vi "Acq 3.5 RT.vi"() -> ()   [LabVIEW 2021]
uses:
  <vilib>/FPGAPlugInAG/myRIO-1900/niLvFpga_Open_myRIO-1900.vi
  <vilib>/rvi/interface/common/dynamic/niFpgaDynamicAddResources.vi
  <vilib>/rvi/interface/common/niFpgaWaitOnOcc.vi
  <vilib>/Utility/error.llb/Error Cluster From Error Code.vi
  <vilib>/rvi/errors/niLvFpgaAdjustHostInterfaceError.vi
  <vilib>/FPGAPlugInAG/Dynamic/niLvFpga_Close_Dynamic.vi
  <vilib>/rvi/interface/nirviOpenFPGA/nirviOpenFPGA.xnode
  FPGA Bitfiles/acquisition3.5co_FPGATarget_Acq3.5FPGA_iMy6CG-4QfE.lvbitx
  <vilib>/rvi/interface/nirviMethod/nirviMethod.xnode
  <vilib>/rvi/interface/nirviReadWriteControl/nirviReadWriteControl.xnode
  <vilib>/rvi/interface/nirviCloseFPGA/nirviCloseFPGA.xnode
  <vilib>/rvi/errors/niLvFpgaMergeErrorWithErrorCode.vi
  <vilib>/FPGAPlugInAG/Dynamic/niLvFpga_ConfigureFifo_Dynamic.vi
  <vilib>/FPGAPlugInAG/Dynamic/niLvFpga_ReadFifo_Dynamic.vi
  <vilib>/FPGAPlugInAG/Dynamic/niLvFpga_StopFifo_Dynamic.vi
  NiFpgaLv.dll
  <vilib>/rvi/interface/Simulation/niFpgaSimulationCallBeginRW.vi
panel:
  out "Loop":i32
  in  "stop":bool
  out "Waveform Graph":waveform(u16)(graph)
  out "Frequency":dbl
  out "Elements Remaing":u32
  in  "Time acq":u32=10
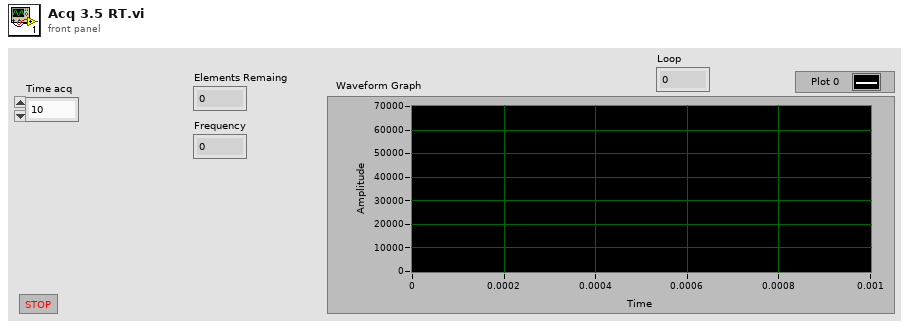
[diagram p1: front panel]
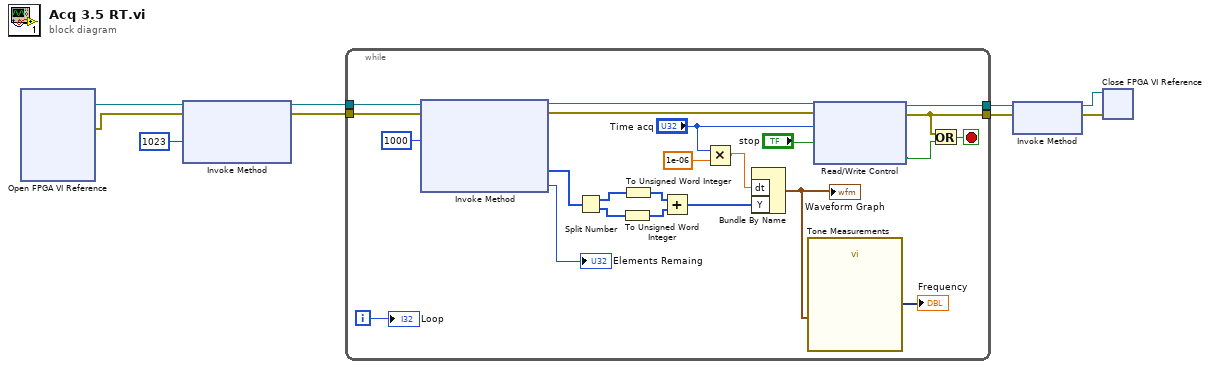
[diagram p0: block diagram]
diagram:
  n1 = xnode "Open FPGA VI Reference"() -> ("FPGA VI Reference Out"=w9:refnum<k20>, "error out"=w8:errorcluster)  [unwired: 2 in]
  n2 = xnode "Invoke Method"("FPGA VI Reference In"=w9, "error in"=w8, "Requested Depth"=u32 1023) -> ("FPGA VI Reference Out"=w6:refnum<k20>, "error out"=w5:errorcluster)  [unwired: 1 out]
  n3 = while {
    tunnel: w6 -> [w31]
    tunnel: w5 -> [w30]
    tunnel: [w16] -> w4
    tunnel: [w15] -> w3
    i -> [w14]
    stop <- w32 stop-if-true
    n4 = xnode "Invoke Method"("FPGA VI Reference In"=w31, "error in"=w30, "Number of Elements"=u32 1000) -> ("FPGA VI Reference Out"=w26:refnum<k20>, "error out"=w25:errorcluster, "Data"=w27:u32[], "Elements Remaining"=→"Elements Remaing":u32)  [unwired: 1 in]
    n5 = Split Number(x=w27) -> (hi(x)=w23:u16[], lo(x)=w22:u16[])
    n6 = To Unsigned Word Integer(number=w22) -> (unsigned 16bit integer=w20:u16[])
    n7 = To Unsigned Word Integer(number=w23) -> (unsigned 16bit integer=w21:u16[])
    n8 = Add(x=w21, y=w20) -> (x+y=w19:u16[])
    n9 = Multiply(x="Time acq", y=1e-06 ("dt")) -> (x*y=w17:dbl)
    n10 = Bundle By Name("dt"=w17, "Y"=w19) -> (w13:waveform(u16))  [unwired: 1 in]
    "Waveform Graph" <- w13
    n11 = call "Tone Measurements"("Signals"=w13) -> ("Frequency"=→"Frequency":dynamicdata)  [unwired: 9 in, 1 out]
    n12 = xnode "Read/Write Control"("FPGA VI Reference In"=w26, "error in"=w25, "Acq Time (us)"="Time acq", "stop"="stop") -> ("FPGA VI Reference Out"=w16:refnum<k20>, "error out"=w15:errorcluster, "stop"=w10:bool)
    n13 = Or(x=w15, y=w10) -> (x .or. y?=w32:bool)
    "Loop" <- w14
  }
  n14 = xnode "Invoke Method"("FPGA VI Reference In"=w4, "error in"=w3) -> ("FPGA VI Reference Out"=w1:refnum<k20>, "error out"=w2:errorcluster)
  n15 = xnode "Close FPGA VI Reference"("FPGA VI Reference In"=w1, "error in"=w2) -> ()  [unwired: 1 out]
